vi "GenerateMoveGeneric.vi"(1 "Input Array":dbl[](array[numeric])) -> (0 "Output":string)   [LabVIEW 2011]
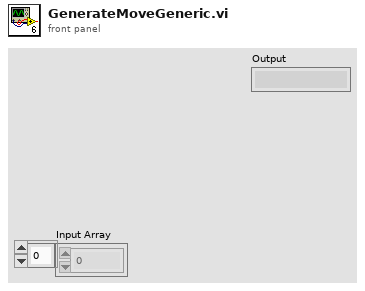
[diagram p1: front panel]
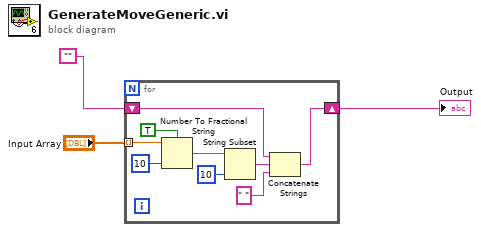
[diagram p0: block diagram]
diagram:
  n1 = for {
    tunnel: "Input Array" -> [w12] mode=indexing
    shift-right: [w4] -> w1
    shift-left: "" -> [w7]
    n2 = Number To Fractional String(use system decimal point (T)=TRUE, number=w12, precision (6)=i16 10) -> (F-format string=w8:string)  [unwired: 1 in]
    n3 = String Subset(string=w8, length (rest)=10 ("length (rest)")) -> (substring=w6:string)  [unwired: 1 in]
    n4 = Concatenate Strings(w7, w6, " " ("F-format string")) -> (w4:string)
  }
  "Output" <- w1
